vi "add_PoseWithCovarianceStamped_roslv.vi"(5 "PoseCovariance":T1={"Pose"={"Point"={"x"=0.0, "y"=0.0, "z"=0.0}, "Quaternion"={"x"=0.0, "y"=0.0, "z"=0.0, "w"=0.0}}, "Covariance"=[0.0, 0.0, 0.0, 0.0, 0.0]}, 6 "Stamp":cluster{"frame_id":string, "reset seq?":bool}, 7 "msg in":string) -> (3 "msg out":string)   [LabVIEW 2014]
doc: "Flattens a pose with covariance stamped into a message"
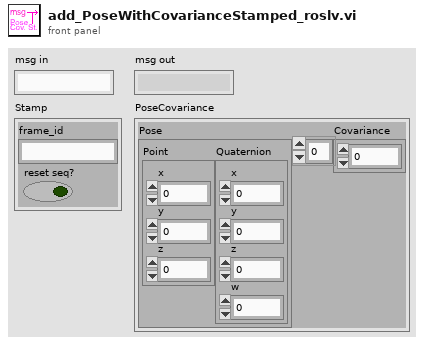
[diagram p1: front panel]
types:
  T1 = cluster{"Pose":cluster{"Point":cluster{"x":dbl, "y":dbl, "z":dbl}, "Quaternion":cluster{"x":dbl, "y":dbl, "z":dbl, "w":dbl}}, "Covariance":dbl[]}
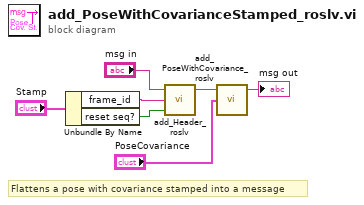
[diagram p0: block diagram]
diagram:
  # "Flattens a pose with covariance stamped into a message"
  n1 = Unbundle By Name("Stamp") -> ("frame_id"=w2:string, "reset seq?"=w1:bool)
  n2 = call "add_Header_roslv.vi"("reset seq?"=w1, "frame_id"=w2, "msg in"="msg in") -> ("msg out"=w6:string)  [unwired: 2 in]
  n3 = call "add_PoseWithCovariance_roslv.vi"("PoseCovariance"="PoseCovariance", "msg in"=w6) -> ("msg out"=→"msg out":string)  [unwired: 3 in]
